vi "niRFUtil FWK Get Dynamic Path.vi"(5 "Virtual Path":path, 7 "Current vi Path":path) -> (8 "Actual Path":path)   [LabVIEW 2015, in "niRFUtil.lvlib"]
uses:
  niRFUtil.lvlib
  <vilib>/regexp/Match Regular Expression.xnode
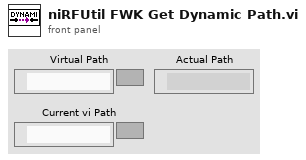
[diagram p1: front panel]
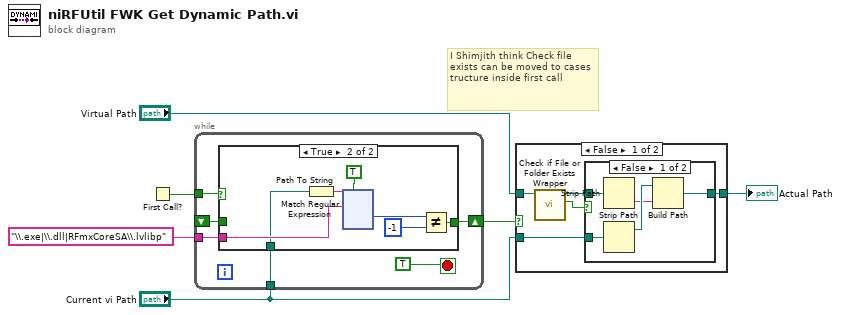
[diagram p0: block diagram]
diagram:
  # "I Shimjith think Check file exists can be moved to cases tructure inside first call"
  n1 = First Call?() -> (First Call?: T/F=w6:bool)
  n2 = while {
    shift-right: [w11] -> w3
    shift-left: _ -> [w10]
    tunnel: w6 -> [w9]
    tunnel: "\\.exe|\\.dll|RFmxCoreSA\\.lvlibp" -> [w8]
    tunnel: "Current vi Path" -> [w7]
    stop <- TRUE stop-if-true
    n3 = case shown="True" w9 {
      tunnel: [w13 w20] -> w11
      tunnel: w10 -> [w13 _]
      tunnel: w8 -> [_ w19]
      tunnel: w7 -> [_ w14]
      frame False {
      }
      frame True {
        n4 = Path To String(path=w14) -> (string=w18:string)
        n5 = xnode "Match Regular Expression"("input string"=w18, "regular expression"=w19, "ignore case? (F)"=TRUE) -> ("offset past match"=w17:i32)  [unwired: 3 in, 4 out]
        n6 = Not Equal?(x=w17, y=-1) -> (x != y?=w20:bool)
      }
    }
  }
  n7 = case shown="False" w3 {
    tunnel: "Virtual Path" -> [w135 w143]
    tunnel: [w134 w143] -> w4
    tunnel: "Current vi Path" -> [w133 _]
    frame False {
      n8 = call "Check if File or Folder Exists Wrapper.vi"("path"=w135) -> ("file or folder exists?"=w132:bool, "dup path"=w136:path)  [unwired: 8 in, 1 out]
      n9 = case shown="False" w132 {
        tunnel: w136 -> [w141 w142]
        tunnel: [w137 w142] -> w134
        tunnel: w133 -> [w140 _]
        frame False {
          n10 = Strip Path(path=w141) -> (name=w138:string)  [unwired: 1 out]
          n11 = Strip Path(path=w140) -> (stripped path=w139:path)  [unwired: 1 out]
          n12 = Build Path(base path=w139, name or relative path=w138) -> (appended path=w137:path)
        }
        frame True {
        }
      }
    }
    frame True {
    }
  }
  "Actual Path" <- w4
